vi "RelativePathToVI.vi"(1 "Relative Path to VI":string, 2 "VI path":path) -> (0 "Absoulte path":path)   [LabVIEW 2020, in "Library Instrument & Equipement.lvlib" / "Library LED Analyser.lvlib"]
doc: "Generates a relative path based on the current VI location"
uses:
  Library LED Analyser.lvlib
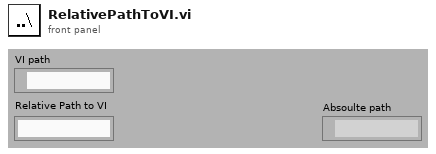
[diagram p1: front panel]
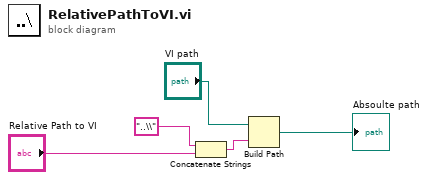
[diagram p0: block diagram]
diagram:
  n1 = Concatenate Strings("..\\", "Relative Path to VI") -> (w5:string)
  n2 = Build Path(base path="VI path", name or relative path=w5) -> (appended path=→"Absoulte path":path)
